vi "Change Selection.vi"(8 "error in (no error)":errorcluster, 10 "UID":string, 11 "Controller in":refnum<class "Controller.lvclass">) -> (0 "error out":errorcluster, 3 "Controller out":refnum<class "Controller.lvclass">)   [LabVIEW 2013, in "SET Project Editor.lvlib" / "Controller.lvclass"]
uses:
  Controller.lvclass
  Controller.lvclass/Controller.ctl
  <vilib>/ActorFramework/Message Enqueuer/Message Enqueuer.lvclass/Message Enqueuer.ctl
  Views/Resource View/Resource View.lvclass
  UI View Messages/Load View to SubPanel Msg/Load View to SubPanel Msg.lvclass/Load View to SubPanel Msg.ctl
  Views/VI List View/VI List View.lvclass
  Views/RTM List View/RTM List View.lvclass
  Views/GObject View/GObject View.lvclass
  Views/VI View/VI View.lvclass
  Views/RTM View/RTM View.lvclass
  Views/Project View/Project View.lvclass
  <vilib>/ActorFramework/Message Enqueuer/Enqueue.vi
  <vilib>/ActorFramework/Message Priority Queue/Priority Enqueue.vi
  <vilib>/ActorFramework/Stop Msg/Stop Msg.lvclass
  UI View Messages/Load View to SubPanel Msg/Load View to SubPanel Msg.lvclass
  SET Project Editor.lvlib
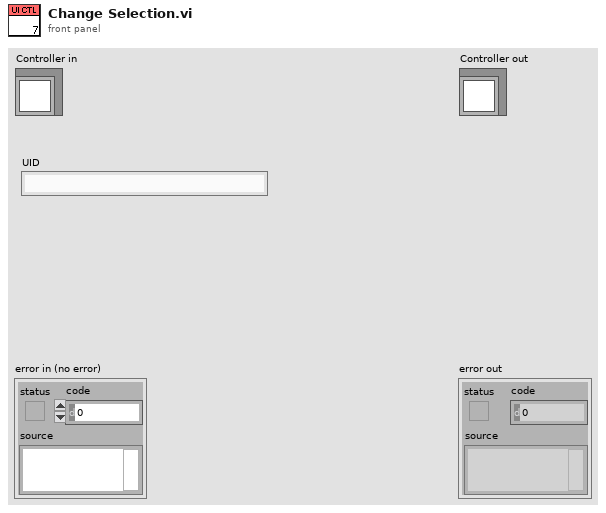
[diagram p1: front panel]
types:
  T1 = typedef "SET Project Editor.lvlib/UID Types.ctl" = enum16{"Invalid", "VI File", "GObject", "GObject Item", "RTM File", "RTM Item"}
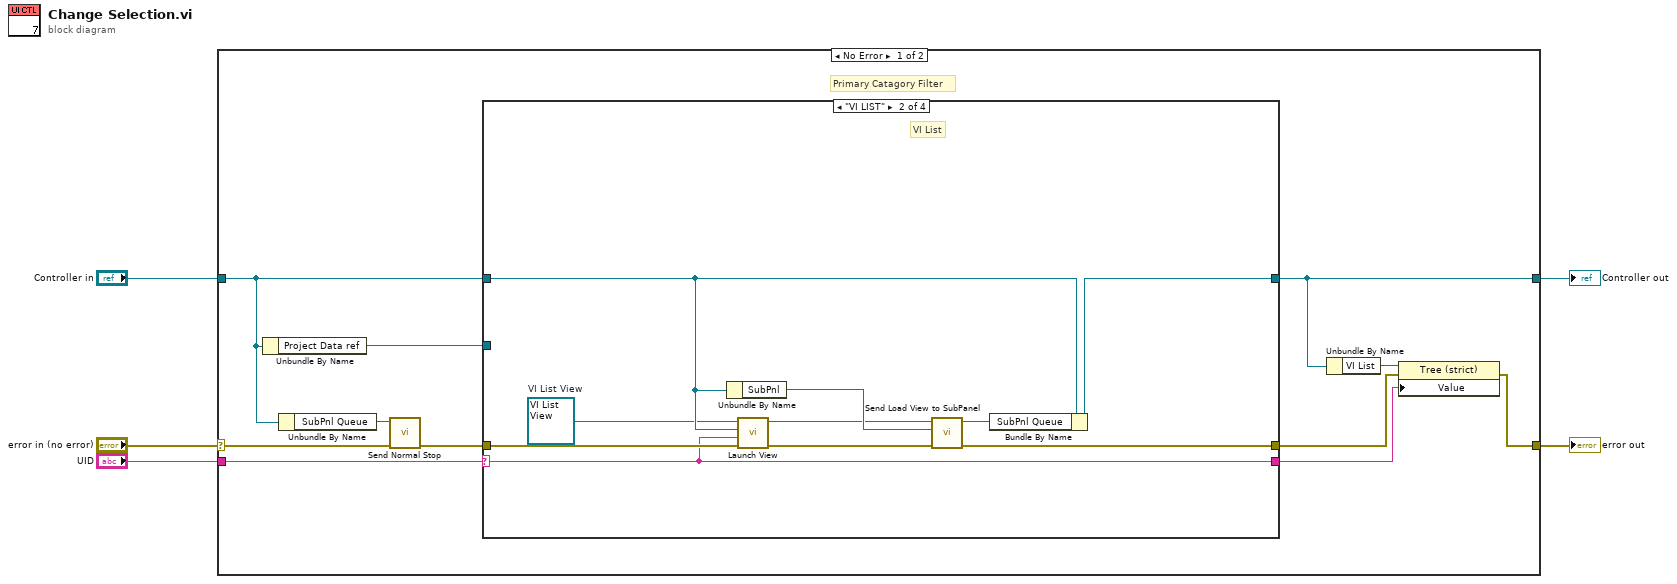
[diagram p0: block diagram]
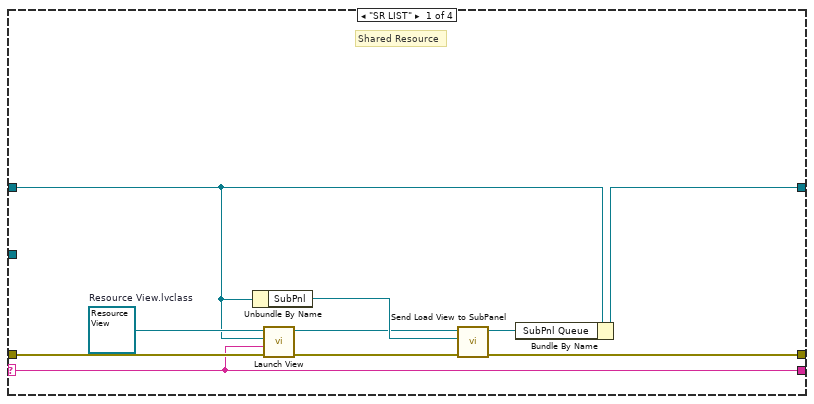
[diagram p2: hidden frame]
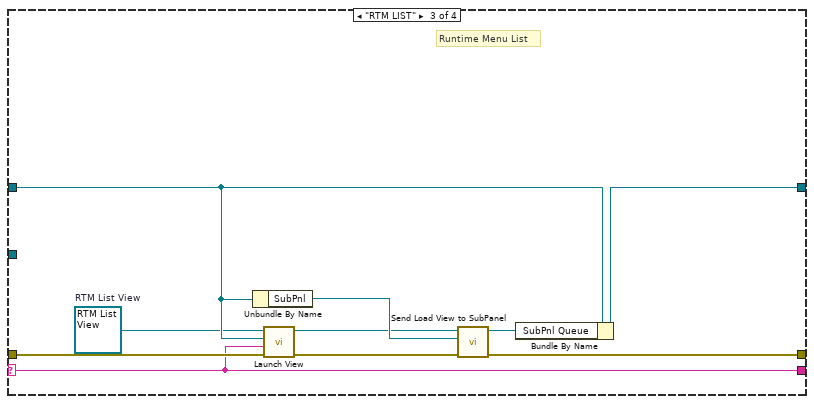
[diagram p3: hidden frame]
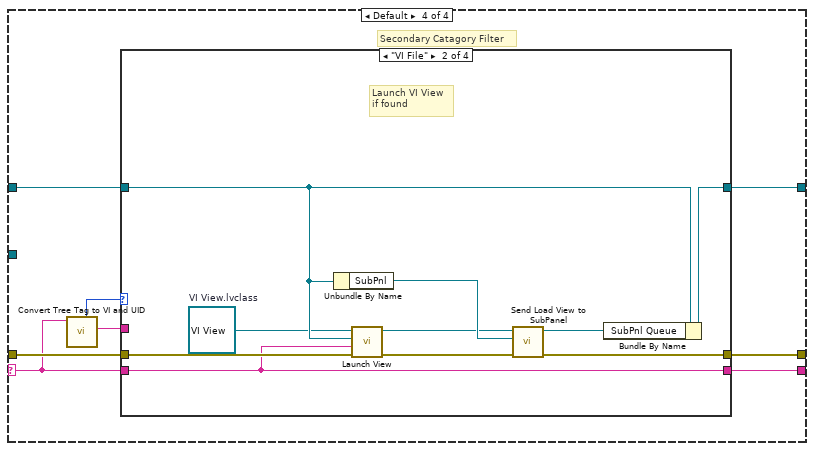
[diagram p4: hidden frame]
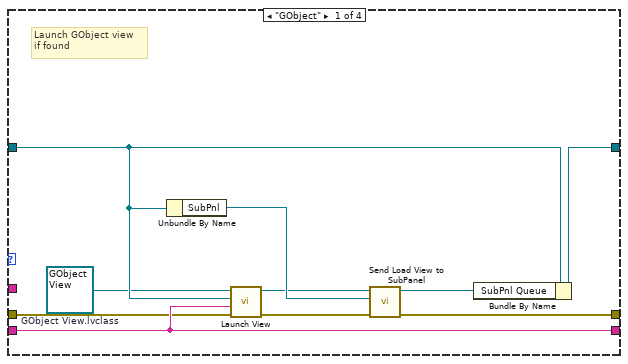
[diagram p5: hidden frame]
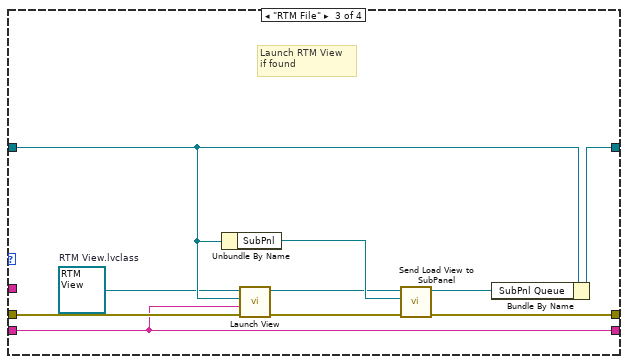
[diagram p6: hidden frame]
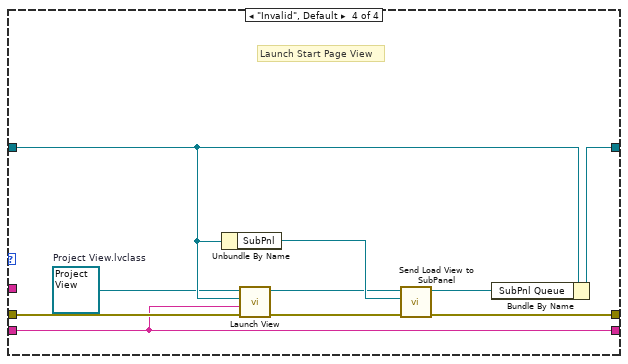
[diagram p7: hidden frame]
diagram:
  n1 = case shown="No Error" "error in (no error)" {
    selector: "error in (no error)" -> [w8 w96]
    tunnel: [w9 w96] -> w4
    tunnel: [w10 w95] -> w2
    tunnel: "Controller in" -> [w14 w95]
    tunnel: "UID" -> [w13 _]
    frame No Error {
      # "Primary Catagory Filter"
      n2 = Unbundle By Name(w14) -> ("Project Data ref"=w12:refnum<data-value>)
      n3 = Unbundle By Name(w14) -> ("SubPnl Queue"=w16:refnum<class "Message Enqueuer.lvclass">)
      n4 = call <vilib>:"Send Normal Stop.vi"("error in (no error)"=w8, "Message Enqueuer"=w16) -> ("error out"=w15:errorcluster)  [unwired: 9 in]
      n5 = case shown="\"VI LIST\"" w13 {
        selector: w13 -> [w17 w28 w38 w50]
        tunnel: w15 -> [w20 w31 w41 w54]
        tunnel: w14 -> [w22 w33 w43 w53]
        tunnel: [w23 w34 w44 w52] -> w10
        tunnel: w12 -> [_ _ _ _]
        tunnel: [w17 w28 w38 w48] -> w7
        tunnel: [w18 w29 w39 w47] -> w6
        frame "SR LIST" {
          w26 = refnum<class "Resource View.lvclass"> refnum  # Resource View.lvclass
          # "Shared Resource"
          n6 = Unbundle By Name(w22) -> ("SubPnl"=w25:refnum<vi>)
          n7 = call-dynamic "Launch View.vi"("error in (no error)"=w20, "UUID"=w17, "Controller in"=w22, "UI View in"=w26) -> ("error out"=w19:errorcluster, "Caller-To-Actor Enqueuer"=w21:refnum<class "Message Enqueuer.lvclass">)  [unwired: 6 in]
          n8 = call "Send Load View to SubPanel.vi"("error in (no error)"=w19, "SubPnl Refnum"=w25, "Message Enqueuer"=w21) -> ("error out"=w18:errorcluster, "Message Enqueuer out"=w24:refnum<class "Message Enqueuer.lvclass">)  [unwired: 7 in]
          n9 = Bundle By Name(cluster=w22, "SubPnl Queue"=w24) -> (w23:refnum<class "Controller.lvclass">)
        }
        frame "VI LIST" {
          w27 = refnum<class "VI List View.lvclass"> refnum  # VI List View
          # "VI List"
          n10 = Unbundle By Name(w33) -> ("SubPnl"=w36:refnum<vi>)
          n11 = call-dynamic "Launch View.vi"("error in (no error)"=w31, "UUID"=w28, "Controller in"=w33, "UI View in"=w27) -> ("error out"=w30:errorcluster, "Caller-To-Actor Enqueuer"=w32:refnum<class "Message Enqueuer.lvclass">)  [unwired: 6 in]
          n12 = call "Send Load View to SubPanel.vi"("error in (no error)"=w30, "SubPnl Refnum"=w36, "Message Enqueuer"=w32) -> ("error out"=w29:errorcluster, "Message Enqueuer out"=w35:refnum<class "Message Enqueuer.lvclass">)  [unwired: 7 in]
          n13 = Bundle By Name(cluster=w33, "SubPnl Queue"=w35) -> (w34:refnum<class "Controller.lvclass">)
        }
        frame "RTM LIST" {
          w37 = refnum<class "RTM List View.lvclass"> refnum  # RTM List View
          # "Runtime Menu List"
          n14 = Unbundle By Name(w43) -> ("SubPnl"=w46:refnum<vi>)
          n15 = call-dynamic "Launch View.vi"("error in (no error)"=w41, "UUID"=w38, "Controller in"=w43, "UI View in"=w37) -> ("error out"=w40:errorcluster, "Caller-To-Actor Enqueuer"=w42:refnum<class "Message Enqueuer.lvclass">)  [unwired: 6 in]
          n16 = call "Send Load View to SubPanel.vi"("error in (no error)"=w40, "SubPnl Refnum"=w46, "Message Enqueuer"=w42) -> ("error out"=w39:errorcluster, "Message Enqueuer out"=w45:refnum<class "Message Enqueuer.lvclass">)  [unwired: 7 in]
          n17 = Bundle By Name(cluster=w43, "SubPnl Queue"=w45) -> (w44:refnum<class "Controller.lvclass">)
        }
        frame Default {
          # "Secondary Catagory Filter"
          n18 = call "Convert Tree Tag to VI and UID.vi"("Tree Tag"=w50) -> ("GObject UID"=w49:string, "UID Type"=w51:T1)  [unwired: 7 in, 2 out]
          n19 = case shown="\"VI File\"" w51 {
            tunnel: w54 -> [w56 w68 w79 w89]
            tunnel: w53 -> [w64 w74 w84 w94]
            tunnel: [w63 w73 w83 w93] -> w52
            tunnel: w50 -> [w57 w65 w76 w86]
            tunnel: w49 -> [_ _ _ _]
            tunnel: [w57 w65 w76 w86] -> w48
            tunnel: [w55 w66 w77 w87] -> w47
            frame "GObject" {
              w62 = refnum<class "GObject View.lvclass"> refnum  # GObject View.lvclass
              # "Launch GObject view\nif found"
              n20 = Unbundle By Name(w64) -> ("SubPnl"=w61:refnum<vi>)
              n21 = call-dynamic "Launch View.vi"("error in (no error)"=w56, "UUID"=w57, "Controller in"=w64, "UI View in"=w62) -> ("error out"=w58:errorcluster, "Caller-To-Actor Enqueuer"=w59:refnum<class "Message Enqueuer.lvclass">)  [unwired: 6 in]
              n22 = call "Send Load View to SubPanel.vi"("error in (no error)"=w58, "SubPnl Refnum"=w61, "Message Enqueuer"=w59) -> ("error out"=w55:errorcluster, "Message Enqueuer out"=w60:refnum<class "Message Enqueuer.lvclass">)  [unwired: 7 in]
              n23 = Bundle By Name(cluster=w64, "SubPnl Queue"=w60) -> (w63:refnum<class "Controller.lvclass">)
            }
            frame "VI File" {
              w72 = refnum<class "VI View.lvclass"> refnum  # VI View.lvclass
              # "Launch VI View\nif found"
              n24 = Unbundle By Name(w74) -> ("SubPnl"=w71:refnum<vi>)
              n25 = call-dynamic "Launch View.vi"("error in (no error)"=w68, "UUID"=w65, "Controller in"=w74, "UI View in"=w72) -> ("error out"=w67:errorcluster, "Caller-To-Actor Enqueuer"=w69:refnum<class "Message Enqueuer.lvclass">)  [unwired: 6 in]
              n26 = call "Send Load View to SubPanel.vi"("error in (no error)"=w67, "SubPnl Refnum"=w71, "Message Enqueuer"=w69) -> ("error out"=w66:errorcluster, "Message Enqueuer out"=w70:refnum<class "Message Enqueuer.lvclass">)  [unwired: 7 in]
              n27 = Bundle By Name(cluster=w74, "SubPnl Queue"=w70) -> (w73:refnum<class "Controller.lvclass">)
            }
            frame "RTM File" {
              w75 = refnum<class "RTM View.lvclass"> refnum  # RTM View.lvclass
              # "Launch RTM View\nif found"
              n28 = Unbundle By Name(w84) -> ("SubPnl"=w82:refnum<vi>)
              n29 = call-dynamic "Launch View.vi"("error in (no error)"=w79, "UUID"=w76, "Controller in"=w84, "UI View in"=w75) -> ("error out"=w78:errorcluster, "Caller-To-Actor Enqueuer"=w80:refnum<class "Message Enqueuer.lvclass">)  [unwired: 6 in]
              n30 = call "Send Load View to SubPanel.vi"("error in (no error)"=w78, "SubPnl Refnum"=w82, "Message Enqueuer"=w80) -> ("error out"=w77:errorcluster, "Message Enqueuer out"=w81:refnum<class "Message Enqueuer.lvclass">)  [unwired: 7 in]
              n31 = Bundle By Name(cluster=w84, "SubPnl Queue"=w81) -> (w83:refnum<class "Controller.lvclass">)
            }
            frame "Invalid", Default {
              w85 = refnum<class "Project View.lvclass"> refnum  # Project View.lvclass
              # "Launch Start Page View"
              n32 = Unbundle By Name(w94) -> ("SubPnl"=w92:refnum<vi>)
              n33 = call-dynamic "Launch View.vi"("error in (no error)"=w89, "UUID"=w86, "Controller in"=w94, "UI View in"=w85) -> ("error out"=w88:errorcluster, "Caller-To-Actor Enqueuer"=w90:refnum<class "Message Enqueuer.lvclass">)  [unwired: 6 in]
              n34 = call "Send Load View to SubPanel.vi"("error in (no error)"=w88, "SubPnl Refnum"=w92, "Message Enqueuer"=w90) -> ("error out"=w87:errorcluster, "Message Enqueuer out"=w91:refnum<class "Message Enqueuer.lvclass">)  [unwired: 7 in]
              n35 = Bundle By Name(cluster=w94, "SubPnl Queue"=w91) -> (w93:refnum<class "Controller.lvclass">)
            }
          }
        }
      }
      n36 = Unbundle By Name(w10) -> ("VI List"=w11:refnum<vi>)
      n37 = property class="Tree (strict)"(reference=w11, error in=w6, "Value"=w7) -> (error out=w9:errorcluster)  [unwired: 1 out]
    }
    frame Error {
    }
  }
  "error out" <- w4
  "Controller out" <- w2
